vi "Simulate Signal to Graph.vi"() -> ()   [LabVIEW 2015]
panel:
  in  "Frequency":dbl(knob) scale=0.0..50.0
  in  "Amplitude":dbl(knob) scale=0.0..10.0
  out "Waveform Chart":dynamicdata(graph)
  in  "stop":bool
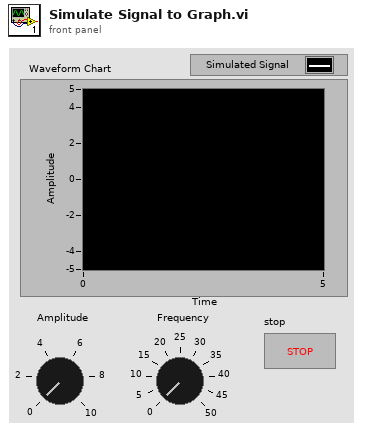
[diagram p1: front panel]
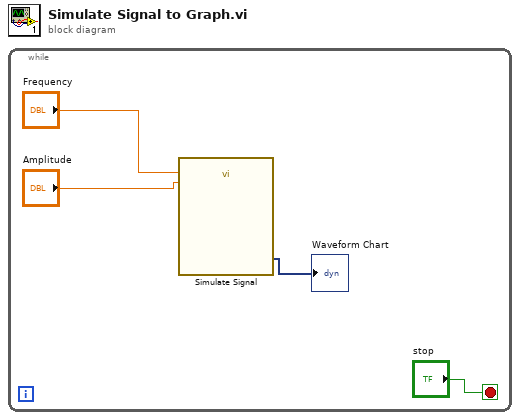
[diagram p0: block diagram]
diagram:
  n1 = while {
    stop <- "stop" stop-if-true
    n2 = call "Simulate Signal"("Frequency"="Frequency", "Amplitude"="Amplitude") -> ("Simulated Signal"=→"Waveform Chart":dynamicdata)  [unwired: 12 in, 1 out]
  }
